vi "ADC_Kernel.vi"(4 "Current Block No":i32, 6 "Sampling rate (Hz)":dbl=1000.0 format="%.2f", 7 "GPIB Address":T5=8, 8 "No of samples":i32=1000, 9 "Local Client?":bool, 10 "Ch & spans":T3[](array[typedef])=[{"high limit (10V)"=10.0, "low limit (-10V)"=-10.0, "Ch No"=0, "Var name"="", "Use Latest Calib"=FALSE}] {"low limit (-10V)" format="%.3f"; "high limit (10V)" format="%.3f"}, 11 "Trigger mode":T2) -> (0 "error out (no error)":errorcluster, 1 "Binary array":i16[][](array[numeric]), 2 "Block Timings":T1={"Started"=0.0, "Ended"=0.0, "Analogue Frequency Hz"=1000.0} {"Analogue Frequency Hz" format="%.2f"}, 3 "group channel settings":T4(array[cluster]) {"scale offset" format="%.2f"; "scale multiplier" format="%.2f"; "gain" format="%.2f"; "range" format="%.2f"; "lower input limits" format="%.2f"; "upper input limits" format="%.2f"}, 5 "Actual Sampling rate (Hz)":dbl=1000.0 format="%.2f")   [LabVIEW 2010]
uses:
  ADC VIs/ADC_GPIB_address.ctl
  Controls/Ch_and_Spans.ctl
  Controls/Trigger_Mode.ctl
  Controls/Block_start_and_end.ctl
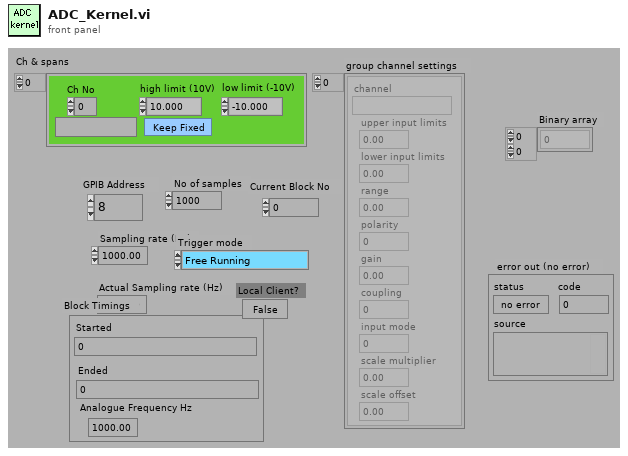
[diagram p1: front panel]
types:
  T1 = typedef "Block_start_and_end.ctl" = cluster{"Started":dbl, "Ended":dbl, "Analogue Frequency Hz":dbl}
  T2 = typedef "Trigger_Mode.ctl" = enum16{"Free Running", "Start on Trigger", "Trigger Every Block", "Trigger Every Sample"}
  T3 = typedef "Ch_and_Spans.ctl" = cluster{"high limit (10V)":sgl, "low limit (-10V)":sgl, "Ch No":i16, "Var name":string, "Use Latest Calib":bool}
  T4 = cluster{"channel":string, "upper input limits":sgl, "lower input limits":sgl, "range":sgl, "polarity":u16, "gain":sgl, "coupling":u16, "input mode":u16, "scale multiplier":dbl, "scale offset":dbl}[]
  T5 = typedef "ADC_GPIB_address.ctl" = u8
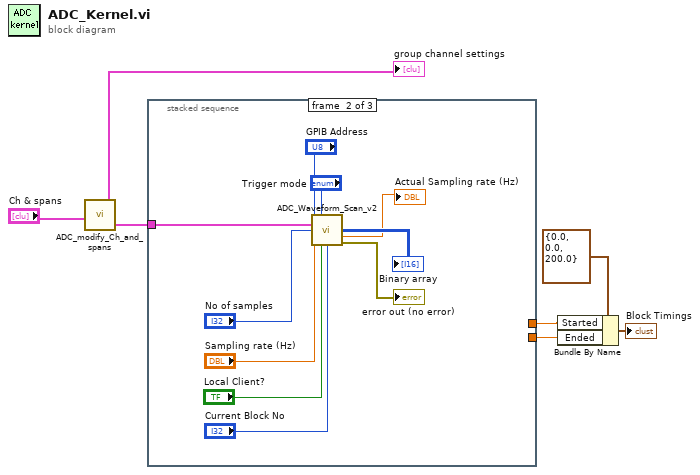
[diagram p0: block diagram]
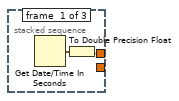
[diagram p2: hidden frame]
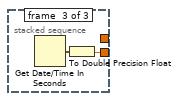
[diagram p3: hidden frame]
diagram:
  n1 = call "ADC_modify_Ch_and_spans.vi"("Ch & spans"="Ch & spans") -> ("group channel settings"=→"group channel settings":T4, "Modified Ch & spans"=w6:T3[])
  n2 = stacked-sequence {
    tunnel: w6 -> [_ w14 _]
    tunnel: [w9 _ _] -> w2
    tunnel: [_ _ w21] -> w1
    frame #0 {
      n3 = Get Date/Time In Seconds() -> (seconds since 1Jan1904=w8:timestamp)
      n4 = To Double Precision Float(number=w8) -> (double precision float=w9:dbl)
    }
    frame #1 {
      n5 = call "ADC_Waveform_Scan_v2.vi"("GPIB Address"="GPIB Address", "Trigger mode"="Trigger mode", "Ch & spans"=w14, "number of scans\n(1000)"="No of samples", "scan rate (1000 scans/sec)"="Sampling rate (Hz)", "Local Client?"="Local Client?", "Current Block No"="Current Block No") -> ("Binary data"=→"Binary array":i16[][], "Actual Sampling rate (Hz)"=→"Actual Sampling rate (Hz)":dbl, "error out"=→"error out (no error)":errorcluster)  [unwired: 2 in, 4 out]
    }
    frame #2 {
      n6 = Get Date/Time In Seconds() -> (seconds since 1Jan1904=w20:timestamp)
      n7 = To Double Precision Float(number=w20) -> (double precision float=w21:dbl)
    }
  }
  n8 = Bundle By Name(cluster=T1 {"Started"=0.0, "Ended"=0.0, "Analogue Frequency Hz"=200.0} ("Block Timings"), "Started"=w2, "Ended"=w1) -> (→"Block Timings":T1)
